vi "copy project and open reference.vi"(8 "error in (no error)":errorcluster, 11 "Builder in":refnum<class "Builder.lvclass">) -> (0 "error out":errorcluster, 3 "Builder out":refnum<class "Builder.lvclass">)   [LabVIEW 2024, in "Builder.lvclass"]
doc: "Copies the project to a random location on Temp folder and open the .lvproj that it finds under ./src folder"
uses:
  builders/parent/Builder.lvclass
  builders/parent/Builder.lvclass/Builder.ctl
  <vilib>/regexp/Match Regular Expression.xnode
  <userlib>/_OpenG.lib/file/file.llb/openg_file.lvlib
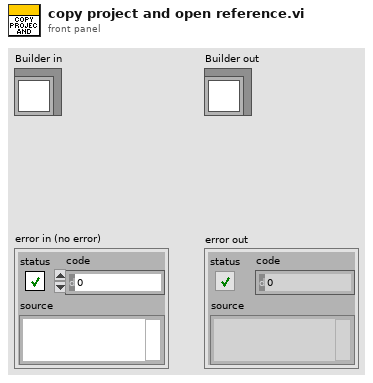
[diagram p1: front panel]
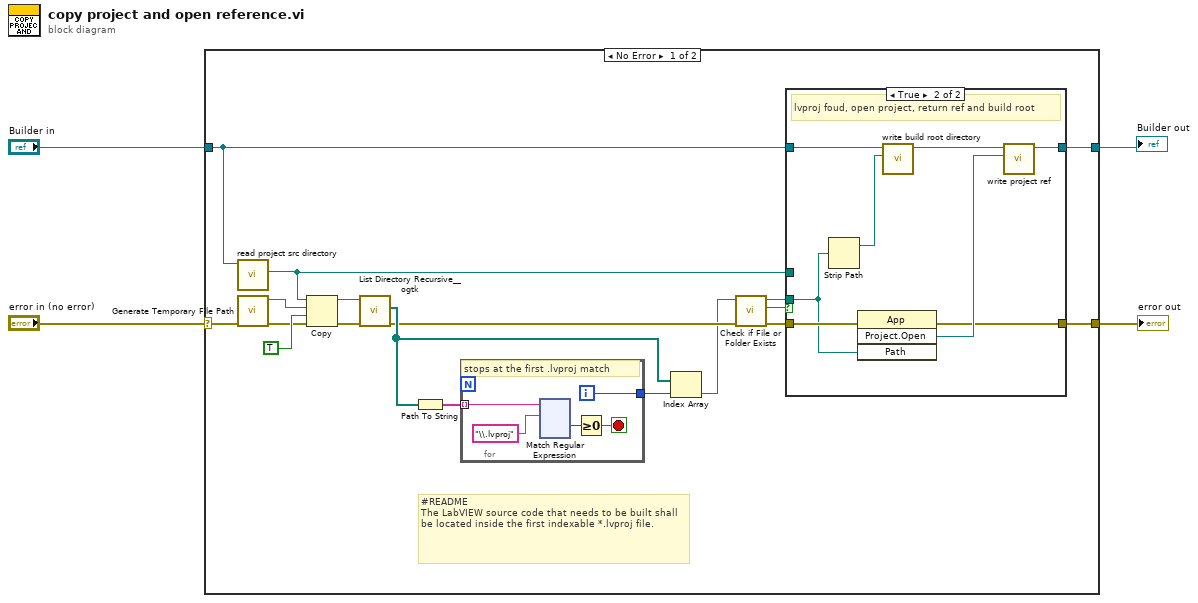
[diagram p0: block diagram]
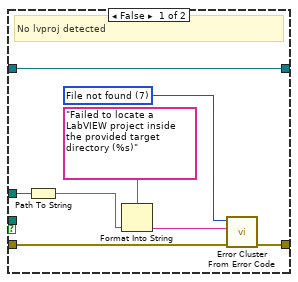
[diagram p2: hidden frame]
diagram:
  n1 = case shown="No Error" "error in (no error)" {
    selector: "error in (no error)" -> [w22 w162]
    tunnel: [w8 w162] -> w4
    tunnel: [w9 w161] -> w2
    tunnel: "Builder in" -> [w6 w161]
    frame No Error {
      # "#README\nThe LabVIEW source code that needs to be built shall be located inside the first indexable *.lvproj file."
      n2 = call "read project src directory.vi"("Builder in"=w6) -> ("project src directory"=w5:path)  [unwired: 10 in]
      n3 = call <vilib>:"Generate Temporary File Path.vi"("error in (no error)"=w22) -> ("error out"=w10:errorcluster, "Unique Temporary File Path"=w12:path)  [unwired: 9 in]
      n4 = Copy(8:w10, 9:TRUE ("overwrite (F)"), 10:w12, 11:w5) -> (0:w20:errorcluster, 3:w21:path)  [unwired: 1 in, 1 out]
      n5 = call <userlib>:"List Directory Recursive__ogtk.vi"("error in (no error)"=w20, "Path"=w21) -> ("error out"=w16:errorcluster, "file paths"=w17:path[])  [unwired: 6 in, 2 out]
      n6 = Path To String(path=w17) -> (string=w19:string[])
      n7 = for {
        tunnel: w19 -> [w43] mode=indexing
        tunnel: [w39] -> w18
        i -> [w39]
        stop <- w41 stop-if-true
        # "stops at the first .lvproj match"
        n8 = xnode "Match Regular Expression"("input string"=w43, "regular expression"="\\.lvproj") -> ("offset past match"=w40:i32)  [unwired: 4 in, 4 out]
        n9 = Greater Or Equal To 0?(x=w40) -> (x >= 0?=w41:bool)
      }
      n10 = Index Array(array=w17, index=w18) -> (element=w14:path)
      n11 = call <vilib>:"Check if File or Folder Exists.vi"("error in (no error)"=w16, "path"=w14) -> ("error out"=w15:errorcluster, "file or folder exists?"=w13:bool, "dup path"=w7:path)  [unwired: 7 in]
      n12 = case shown="True" w13 {
        tunnel: w15 -> [w30 w38]
        tunnel: w6 -> [w28 w36]
        tunnel: [w28 w35] -> w9
        tunnel: [w29 w34] -> w8
        tunnel: w5 -> [w27 _]
        tunnel: w7 -> [_ w31]
        frame False {
          w26 = 7 items=["No error", "Argument error", "Memory is full", "Out of zone", "End of file", "File already open", "Generic file I/O error", "File not found", "File permission error", "Disk is full", "Duplicate path", "Too many files open", "System feature not enabled", "Resource file not found", "Cannot add resource", "Resource not found", "Image not found", "Image memory error", "Pen does not exist", "Config type invalid", "Config token not found", "Config parse error", "Config memory error", "Bad external code format", "Bad external code offset", "External code not present", "Null window", "Destroy window error", "Null menu", "Print aborted", "Bad print record", "Print driver error", "Windows error during printing", "Memory error during printing", "Print dialog error", "Generic print error", "Invalid device refnum", "Device not found", "Device parameter error", "Device unit error", "Cannot open device", "Device call aborted", "Generic error", "Cancelled by user", "Object ID too low", "Object ID too high", "Object not in heap", "Unknown heap", "Unknown object (invalid DefProc)", "Unknown object (DefProc not in table)", "Message out of range", "Invalid (null) method", "Unknown message", "Manager call not supported", "Bad address", "Network operation in progress", "Network operation timed out", "Connection is busy", "Network attribute not supported", "Network error", "Address in use", "System out of memory", "Connection aborted", "Connection refused", "Not connected", "Already connected", "Connection closed", "Initialization error (interapplication manager)", "Bad occurrence", "Wait on unbound occurrence handler", "Occurrence queue overflow", "Datalog type conflict", "Unused", "Unrecognized type (interapplication manager)", "Memory corrupt", "Failed to make temporary DLL", "Old CIN version", "Drag socket not found", "Failed to load drop-object", "Failed to register OLE object", "Failed to release OLE object", "Format specifier type mismatch", "Unknown format specifier", "Too few format specifiers", "Too many format specifiers", "Scan failed", "Newer CIN version", "Error converting to variant", "Runtime menu error", "Password tampered", "Variant attribute not found", "Incompatible variant data type", "Event data is not available", "Event Store is not present", "Occurrence is not found", "Event Queue is not created", "Event info is not available", "Refnum passed is NULL", "Error retrieving Class GUID", "Error retrieving CoClass GUID", "Error retrieving TypeLib GUID.", "Bad built application magic bytes.", "Specific driver is different from the specific driver associated with the Logical Name.", "There is no session opened to the class driver.", "Max Error", "MAX - Error with config objects", "MAX - Error loading configuration", "MAX - Group not supported"]
          # "No lvproj detected"
          n13 = Path To String(path=w27) -> (string=w23:string)
          n14 = Format Into String(format string="Failed to locate a LabVIEW project inside the provided target directory (%s)", w23) -> (resulting string=w24:string)  [unwired: 2 in, 1 out]
          n15 = call <vilib>:"Error Cluster From Error Code.vi"("error in (no error)"=w30, "error message (\"\")"=w24, "error code (0)"=w26) -> ("error out"=w29:errorcluster)  [unwired: 6 in]
        }
        frame True {
          # "lvproj foud, open project, return ref and build root"
          n16 = Strip Path(path=w31) -> (stripped path=w32:path)  [unwired: 1 out]
          n17 = invoke class="App" method="Project.Open"(error in=w38, "Path"=w31) -> (error out=w34:errorcluster, "Project:Open"=w37:refnum<vi>)  [unwired: 2 in, 2 out]
          n18 = call "write build root directory.vi"("build root directory"=w32, "Builder in"=w36) -> ("Builder out"=w33:refnum<class "Builder.lvclass">)  [unwired: 9 in]
          n19 = call "write project ref.vi"("project ref"=w37, "Builders in"=w33) -> ("Builders out"=w35:refnum<class "Builder.lvclass">)  [unwired: 9 in]
        }
      }
    }
    frame Error {
    }
  }
  "error out" <- w4
  "Builder out" <- w2
